vi "VCI Get Reference.vi"(6 "pData":u32, 7 "RefType":u32, 9 "CANIndex":u32, 10 "DevIndex":u32, 11 "DevType":u32) -> (3 "function return":u32, 4 "pData out":u32)   [LabVIEW 2010, in "ControlCAN.lvlib"]
doc: "unsigned int WINAPI VCI_GetReference(unsigned int DevType,unsigned int DevIndex,unsigned int CANIndex,unsigned int RefType,void *pData);"
uses:
  ControlCAN.lvlib
  ControlCAN/Ginkgo_Driver.dll
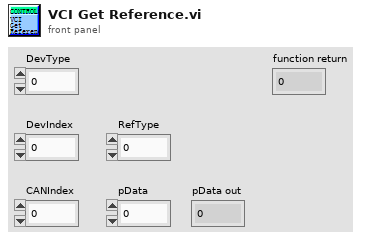
[diagram p1: front panel]
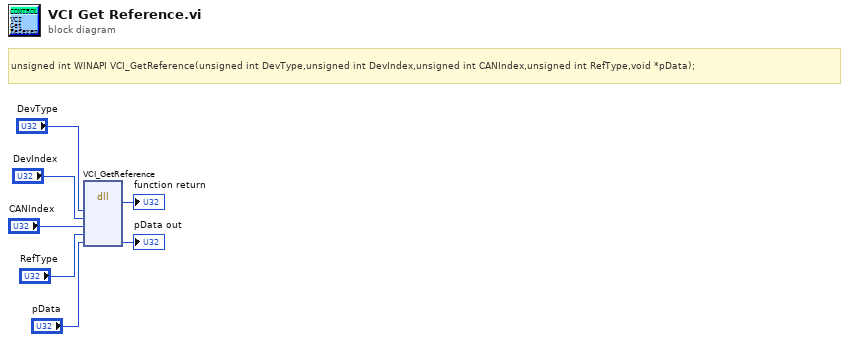
[diagram p0: block diagram]
diagram:
  # "unsigned int WINAPI VCI_GetReference(unsigned int DevType,unsigned int DevIndex,unsigned int CANIndex,unsigned int RefType,void *pData);"
  n1 = dll-call lib="E:/Project/vt_ginkgo/truck/Ginkgo Driver/vs2010/Ginkgo_USB-I2C&SPI&CAN_API_v2.0.3.3/lib/labview_32bit/ControlCAN/Ginkgo_Driver.*" fn="VCI_GetReference"("DevType"="DevType", "DevIndex"="DevIndex", "CANIndex"="CANIndex", "RefType"="RefType", "pData"="pData") -> (→"function return":u32, "pData"=→"pData out":u32)  [unwired: 7 in, 2 out]
